vi "RTS Read Door Setup.vi"(8 "Error In":errorcluster, 10 "Data Out":T1) -> (0 "Error Out":errorcluster, 2 "Read Door CMD":string)   [LabVIEW 2016]
uses:
  Type Definitions/RTS TCP Multiple Connections Data.ctl
  <vilib>/Utility/error.llb/whitespace.ctl
  Type Definitions/RTS TCP Commands.ctl
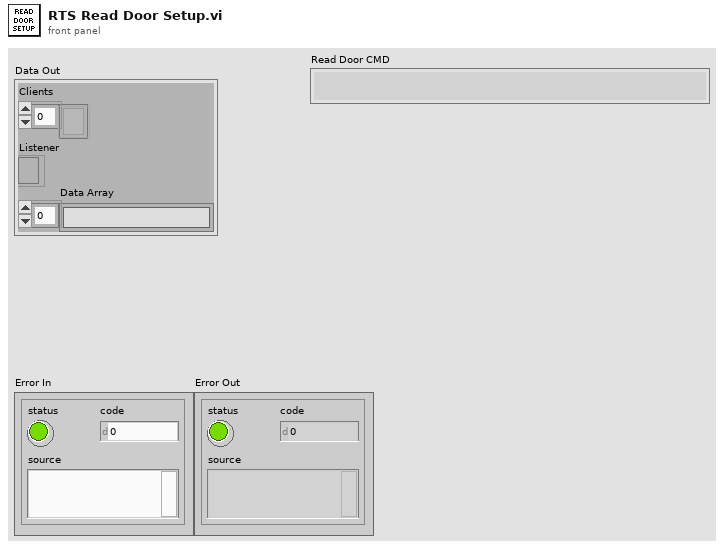
[diagram p1: front panel]
types:
  T1 = typedef "RTS TCP Multiple Connections Data.ctl" = cluster{"Clients":refnum<k5>[], "Listener":refnum<k5>, "Data Array":string[]}
  T2 = typedef "whitespace.ctl" = u16
  T3 = typedef "RTS TCP Commands.ctl" = string
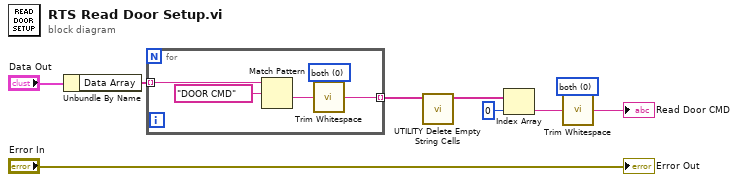
[diagram p0: block diagram]
diagram:
  w1 = T2 0 items=["both", "start of string", "end of string"] ("location (both)")
  n1 = Unbundle By Name("Data Out") -> ("Data Array"=w7:string[])
  n2 = for {
    tunnel: w7 -> [w14] mode=indexing
    tunnel: [w11] -> w5 mode=indexing
    w10 = T2 0 items=["both", "start of string", "end of string"] ("location (both)")
    n3 = Match Pattern(string=w14, regular expression=T3 "DOOR CMD" ("TCP Commands")) -> (after substring=w12:string)  [unwired: 1 in, 3 out]
    n4 = call <vilib>:"Trim Whitespace.vi"("string"=w12, "location (both)"=w10) -> ("trimmed string"=w11:string)
  }
  n5 = call "UTILITY Delete Empty String Cells.vi"("Array with Empty Cells"=w5) -> ("Array w/o Empty Cells"=w4:string[])  [unwired: 10 in]
  n6 = Index Array(array=w4, index=0) -> (element=w3:string)
  n7 = call <vilib>:"Trim Whitespace.vi"("string"=w3, "location (both)"=w1) -> ("trimmed string"=→"Read Door CMD":string)
  "Error Out" <- "Error In"
